vi "Write ISDAFactory.vi"(10 "ISDAFactory.lvclass":refnum<class "ISDAFactory.lvclass">, 11 "Model in":refnum<class "Model.lvclass">) -> (3 "Model out":refnum<class "Model.lvclass">)   [LabVIEW 2013, in "Model.lvclass"]
uses:
  Model.lvclass
  ISDAFactory/ISDAFactory.lvclass
  Model.lvclass/Model.ctl
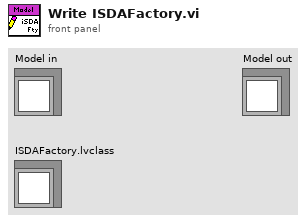
[diagram p1: front panel]
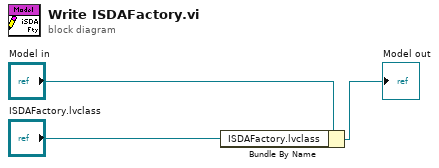
[diagram p0: block diagram]
diagram:
  n1 = Bundle By Name(cluster="Model in", "ISDAFactory.lvclass"="ISDAFactory.lvclass") -> (→"Model out":refnum<class "Model.lvclass">)
